vi "Replace Illegal Characters.vi"(1 "Replacement Character (_)":string="_", 2 "Illegal Character List (/\\:*?\"<>|)":string[](array[string])=["/", "\\", ":", "*", "?", "\"", "<", ">", "|"], 3 "String":string) -> (0 "Output String":string)   [LabVIEW 2018]
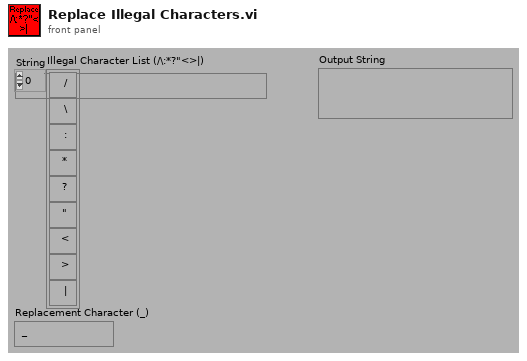
[diagram p1: front panel]
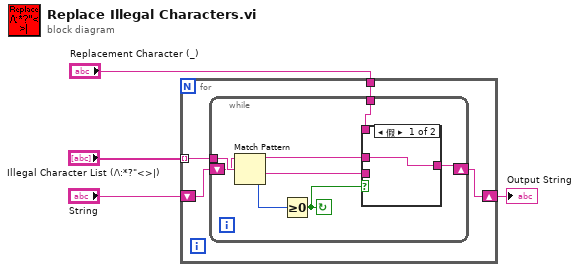
[diagram p0: block diagram]
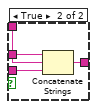
[diagram p2: hidden frame]
diagram:
  n1 = for {
    tunnel: "Illegal Character List (/\\:*?\"<>|)" -> [w8] mode=indexing
    shift-right: [w6] -> w1
    shift-left: "String" -> [w7]
    tunnel: "Replacement Character (_)" -> [w5]
    n2 = while {
      tunnel: w5 -> [w9]
      shift-left: w7 -> [w15]
      shift-right: [w12] -> w6
      tunnel: w8 -> [w16]
      stop <- w10 continue-if-true
      n3 = Match Pattern(string=w15, regular expression=w16) -> (before substring=w14:string, after substring=w13:string, offset past match=w11:i32)  [unwired: 1 in, 1 out]
      n4 = Greater Or Equal To 0?(x=w11) -> (x >= 0?=w10:bool)
      n5 = case shown="假" w10 {
        tunnel: w14 -> [w17 w21]
        tunnel: w13 -> [_ w20]
        tunnel: [w17 w19] -> w12
        tunnel: w9 -> [_ w18]
        frame False {
        }
        frame True {
          n6 = Concatenate Strings(w21, w18, w20) -> (w19:string)
        }
      }
    }
  }
  "Output String" <- w1
